vi "GetDataForExcel.FillClust.vi"(7 "Type":u16, 8 "error in":errorcluster, 11 "path":path) -> (0 "error out":errorcluster, 2 "Array":string[](array[string]), 3 "path out":path)   [LabVIEW 2013, in "main.lvlib"]
uses:
  main.lvlib
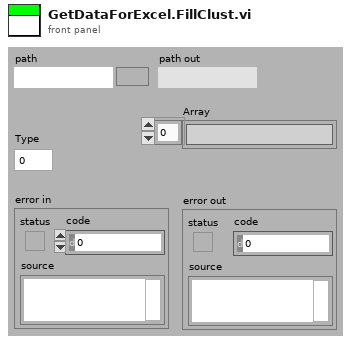
[diagram p1: front panel]
types:
  T1 = cluster{"Over Knæ":string, "Under Knæ":string, "Ankel":string, "Hæl":string, "Forfod":string, "Tå":string, "Yderligere":string}
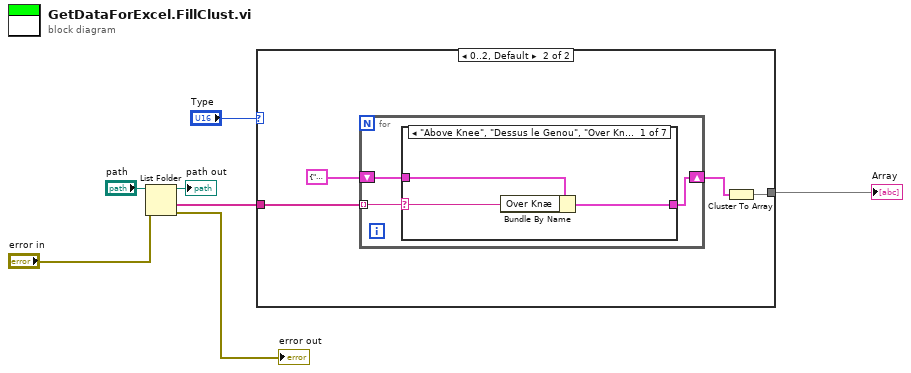
[diagram p0: block diagram]
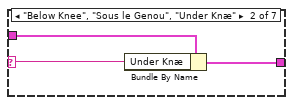
[diagram p3: hidden frame]
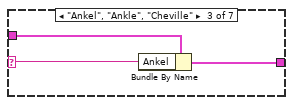
[diagram p4: hidden frame]
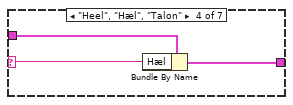
[diagram p5: hidden frame]
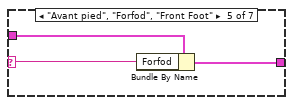
[diagram p6: hidden frame]
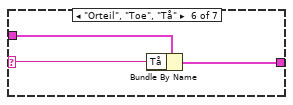
[diagram p7: hidden frame]
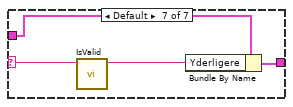
[diagram p8: hidden frame]
diagram:
  n1 = List Folder(path="path", error in="error in") -> (path out=→"path out":path, folder names=w5:string[], error out=→"error out":errorcluster)  [unwired: 2 in, 1 out]
  n2 = case shown="0..2, Default" "Type" {
    tunnel: w5 -> [w8 w11]
    tunnel: [w8 w9] -> w6
    frame 3 {
    }
    frame 0..2, Default {
      n3 = for {
        tunnel: w11 -> [w15] mode=indexing
        shift-right: [w14] -> w10
        shift-left: T1 {"Over Knæ"="", "Under Knæ"="", "Ankel"="", "Hæl"="", "Forfod"="", "Tå"="", "Yderligere"=""} -> [w13]
        n4 = case shown="\"Above Knee\", \"Dessus le Genou\", \"Over Knæ\"" w15 {
          selector: w15 -> [w18 w19 w22 w25 w28 w31 w35]
          tunnel: [w17 w20 w23 w26 w29 w32 w36] -> w14
          tunnel: w13 -> [w16 w21 w24 w27 w30 w33 w37]
          frame "Above Knee", "Dessus le Genou", "Over Knæ" {
            n5 = Bundle By Name(cluster=w16, "Over Knæ"=w18) -> (w17:T1)
          }
          frame "Below Knee", "Sous le Genou", "Under Knæ" {
            n6 = Bundle By Name(cluster=w21, "Under Knæ"=w19) -> (w20:T1)
          }
          frame "Ankel", "Ankle", "Cheville" {
            n7 = Bundle By Name(cluster=w24, "Ankel"=w22) -> (w23:T1)
          }
          frame "Heel", "Hæl", "Talon" {
            n8 = Bundle By Name(cluster=w27, "Hæl"=w25) -> (w26:T1)
          }
          frame "Avant pied", "Forfod", "Front Foot" {
            n9 = Bundle By Name(cluster=w30, "Forfod"=w28) -> (w29:T1)
          }
          frame "Orteil", "Toe", "Tå" {
            n10 = Bundle By Name(cluster=w33, "Tå"=w31) -> (w32:T1)
          }
          frame Default {
            n11 = call "IsValid.vi"("String"=w35) -> ("String 2"=w34:string)  [unwired: 10 in]
            n12 = Bundle By Name(cluster=w37, "Yderligere"=w34) -> (w36:T1)
          }
        }
      }
      n13 = Cluster To Array(cluster=w10) -> (array=w9:string[])
    }
  }
  "Array" <- w6
